vi "CRC32.vi"(11 "ByteArrayIn":u8[](array[numeric])) -> (0 "CRCByteArray":u8[](array[numeric]), 3 "CRC":u32 format="%08x")   [LabVIEW 2016, in "FPGAMockGyro.lvlib"]
doc: "Calculates a 32-bit CRC. The default is the CRC-32-IEEE 802.3 with the following parameters:\n Polynomial - 0xEDB88320\n Initial CRC - 0xFFFFFFFF\n Final XOR Value - 0xFFFFFFFF\n Reflect Input - TRUE\n Reflect CRC - TRUE"
uses:
  FPGAMockGyro.lvlib
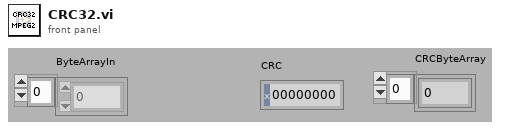
[diagram p1: front panel]
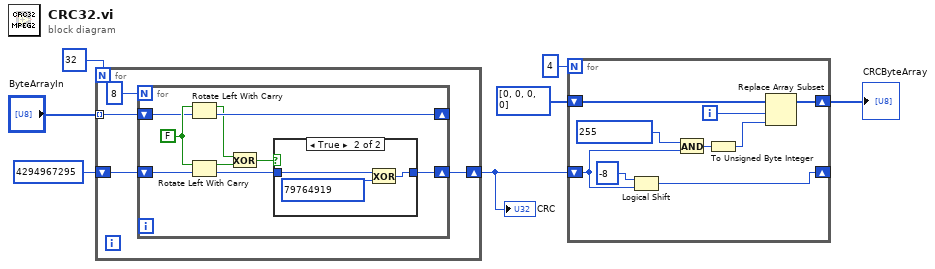
[diagram p0: block diagram]
diagram:
  n1 = for {
    N: 32 -> [_]
    shift-right: [w8] -> w3
    shift-left: u32 4294967295 ("Initial CRC") -> [w10]
    tunnel: "ByteArrayIn" -> [w9] mode=indexing
    n2 = for {
      N: 8 -> [_]
      shift-right: [w15] -> w8
      shift-left: w10 -> [w13]
      shift-right: [w18] -> _
      shift-left: w9 -> [w19]
      w20 = FALSE ("carry")
      n3 = Rotate Left With Carry(2:w19, 3:w20) -> (0:w18:u8, 1:w17:bool)
      n4 = Rotate Left With Carry(2:w13, 3:w20) -> (0:w12:u32, 1:w14:bool)
      n5 = Exclusive Or(1:w14, 2:w17) -> (0:w16:bool)
      n6 = case shown="True" w16 {
        tunnel: w12 -> [w21 w24]
        tunnel: [w21 w23] -> w15
        frame False {
        }
        frame True {
          n7 = Exclusive Or(1:u32 79764919, 2:w24) -> (0:w23:u32)
        }
      }
    }
  }
  "CRC" <- w3
  n8 = for {
    N: 4 -> [_]
    shift-right: [w29] -> _
    shift-left: w3 -> [w31]
    shift-right: [w27] -> w2
    shift-left: u8[] [0, 0, 0, 0] -> [w26]
    i -> [w25]
    n9 = Logical Shift(y=i16 -8, x=w31) -> (x << y=w29:u32)
    n10 = And(x=u32 255, y=w31) -> (x .and. y?=w32:u32)
    n11 = To Unsigned Byte Integer(number=w32) -> (unsigned 8bit integer=w28:u8)
    n12 = Replace Array Subset(array=w26, new element=w28, index=w25) -> (w27:u8[])
  }
  "CRCByteArray" <- w2
